vi "L0_Sum.vi"() -> ()   [LabVIEW 2012]
uses:
  <vilib>/Utility/file.llb/Write To Spreadsheet File (string).vi
panel:
  in  "Atenuation":i32[](array[numeric])=[0, 4, 8, 12]
  out "Clip Index":i32=3
  out "Attenuation":i32=12
  out "Ib Clipping\nLevel":i32=63
  in  "Ib Clipping":i32[](array[numeric])=[1, 16, 32, 64, 32, 40, 48, 56, 63]
  out "Delay Line\n(Asic Chan.)":i32=5
  out "VISA resource name out":refnum<visa-resource-name>
  out "error 2 out":errorcluster={"status"=TRUE, "code"=-1073807202, "source"="VISA Open in Agilent 81150.lvlib:Initialize.vi->Set_Gen_Conf.vi->L0_ClippingNDiscrim.vi"}
  in  "error in 1":errorcluster
  in  "Osc":refnum<visa-resource-name>="Oscilloscope"
  in  "Generator":refnum<visa-resource-name>="generadorpulsos"
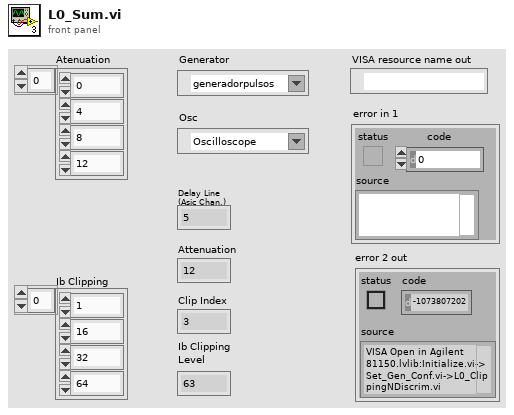
[diagram p1: front panel]
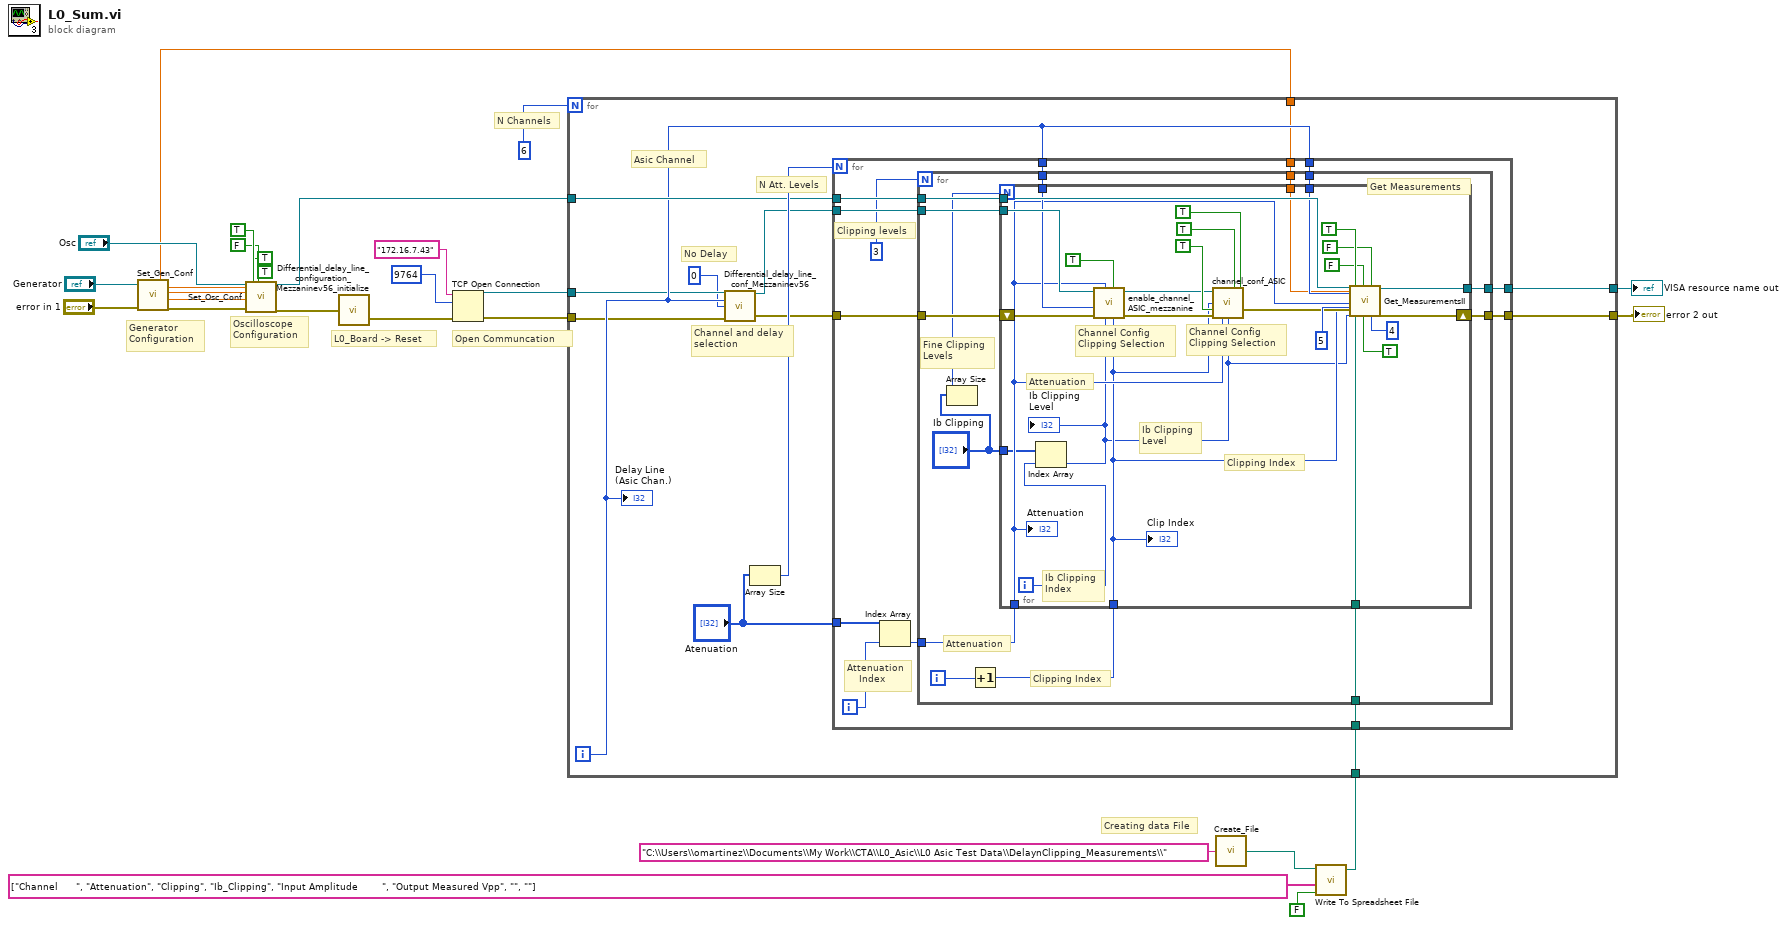
[diagram p0: block diagram]
diagram:
  # "Creating data File"
  # "Open Communcation"
  # "Oscilloscope\nConfiguration"
  # "Generator \nConfiguration"
  # "N Channels"
  # "L0_Board -> Reset"
  n1 = call "Set_Gen_Conf.vi"("AWG VISA"="Generator", "error in (no error)"="error in 1") -> ("Amplitude 1 OUT"=w1:dbl, "Pulse Width in seconds 1 OUT"=w10:dbl, "Trigger Level 1"=w11:dbl, "error out"=w18:errorcluster)  [unwired: 10 in, 4 out]
  n2 = call "Set_Osc_Conf.vi"("VISA resource name"="Osc", "Amplitude IN"=w1, "Trigger Level IN"=w11, "Pulse Width in seconds IN"=w10, "error in (no error)"=w18, "Channel 1"=TRUE, "Channel 3"=TRUE, "Channel 2"=FALSE, "Channel 4"=TRUE) -> ("VISA resource name out"=w6:refnum<visa-resource-name>, "error out"=w17:errorcluster)  [unwired: 9 in]
  n3 = call "Differential_delay_line_configuration_Mezzaninev56_initialize.vi"("error in (no error)"=w17) -> ("error out 2"=w14:errorcluster)  [unwired: 1 in]
  n4 = TCP Open Connection(address="172.16.7.43", remote port or service name=u16 9764, error in (no error)=w14) -> (connection ID=w5:refnum<k5>, error out=w4:errorcluster)  [unwired: 2 in]
  n5 = call "Create_File.vi"("String"="C:\\Users\\omartinez\\Documents\\My Work\\CTA\\L0_Asic\\L0 Asic Test Data\\DelaynClipping_Measurements\\") -> ("path"=w12:path)
  n6 = call-poly <vilib>:"Write To Spreadsheet File.vi"("append to file? (new file:F)"=FALSE, "1D data"=string[] ["Channel      ", "Attenuation", "Clipping", "Ib_Clipping", "Input Amplitude        ", "Output Measured Vpp", "", ""], "file path (dialog if empty)"=w12) -> ("new file path (Not A Path if cancelled)"=w2:path)  [unwired: 5 in]
  n7 = for {
    N: 6 -> [_]
    tunnel: w5 -> [w32]
    tunnel: w4 -> [w33]
    tunnel: w6 -> [w35]
    tunnel: [w29] -> w9
    tunnel: [w30] -> w8
    tunnel: w2 -> [w31]
    tunnel: w1 -> [w27]
    i -> [w34]
    # "No Delay"
    # "Asic Channel"
    # "N Att. Levels"
    # "Channel and delay\nselection"
    n8 = call "Differential_delay_line_conf_Mezzaninev56.vi"("connection ID"=w32, "channel"=w34, "Delay value"=0, "error in (no error)"=w33) -> ("connection ID out"=w36:refnum<k5>, "error out 2"=w37:errorcluster)  [unwired: 4 in, 6 out]
    n9 = Array Size(array="Atenuation") -> (size(s)=w38:i32)
    n10 = for {
      N: w38 -> [_]
      tunnel: w36 -> [w52]
      tunnel: w35 -> [w51]
      tunnel: w37 -> [w50]
      tunnel: "Atenuation" -> [w48]
      tunnel: w34 -> [w45]
      tunnel: w31 -> [w44]
      tunnel: w34 -> [w43]
      tunnel: [w42] -> w29
      tunnel: [w41] -> w30
      tunnel: w27 -> [w40]
      i -> [w47]
      # "Clipping levels"
      # "Attenuation\n    Index"
      n11 = Index Array(array=w48, index=w47) -> (element=w46:i32)
      n12 = for {
        N: 3 -> [_]
        tunnel: w52 -> [w66]
        tunnel: w51 -> [w65]
        tunnel: w50 -> [w64]
        tunnel: w46 -> [w61]
        tunnel: w45 -> [w62]
        tunnel: w44 -> [w59]
        tunnel: w43 -> [w58]
        tunnel: [w57] -> w42
        tunnel: [w56] -> w41
        tunnel: w40 -> [w53]
        i -> [w63]
        # "Get Measurements"
        # "Fine Clipping\nLevels"
        # "Attenuation"
        # "Clipping Index"
        n13 = Array Size(array="Ib Clipping") -> (size(s)=w55:i32)
        n14 = Increment(x=w63) -> (x+1=w60:i32)
        n15 = for {
          N: w55 -> [_]
          tunnel: w66 -> [w90]
          tunnel: w65 -> [w86]
          tunnel: w61 -> [w74]
          tunnel: w62 -> [w84]
          tunnel: w60 -> [w73]
          tunnel: w59 -> [w82]
          tunnel: w58 -> [w80]
          tunnel: [w77] -> w56
          shift-right: [w78] -> w57
          shift-left: w64 -> [w85]
          tunnel: "Ib Clipping" -> [w72]
          tunnel: w53 -> [w69]
          i -> [w70]
          # "Channel Config\nClipping Selection"
          # "Clipping Index"
          # "Ib Clipping\nLevel"
          # "Attenuation"
          # "Ib Clipping\nIndex"
          # "Channel Config\nClipping Selection"
          n16 = Index Array(array=w72, index=w70) -> (element=w71:i32)
          "Ib Clipping\nLevel" <- w71
          n17 = call "enable_channel_ASIC_mezzanine.vi"("Clip_sel_b"=w73, "maj/sum"=TRUE, "Ib_clipVb"=w71, "Att gain"=w74, "error in"=w85, "Channel"=w84, "connection ID"=w90) -> ("error out"=w91:errorcluster, "connection ID out"=w89:refnum<k5>)  [unwired: 2 in, 1 out]
          n18 = call "channel_conf_ASIC.vi"("connection ID"=w89, "Clip_sel_b"=w73, "CompBuf_en_b"=TRUE, "error out"=w91, "Att gain"=w74, "Ib_ClipVb"=w71, "Clip_en_b"=TRUE, "Att_en_b"=TRUE) -> ("error out 2"=w75:errorcluster)  [unwired: 3 in, 4 out]
          n19 = call "Get_MeasurementsII.vi"("VISA resource name"=w86, "Amplitude IN"=w69, "Attenuation"=w74, "Measurements per channel"=5, "Clipping"=w73, "Fine Clipping"=w71, "Amplitude"=TRUE, "file path (dialog if empty)"=w82, "Width"=FALSE, "Write to a file?"=TRUE, "ASIC Channel"=w80, "error in"=w75, "Delay"=FALSE, "Oscilloscope Channel"=4) -> ("VISA resource name out"=w77:refnum<visa-resource-name>, "error out"=w78:errorcluster)  [unwired: 9 in, 3 out]
          "Clip Index" <- w73
          "Attenuation" <- w74
        }
      }
    }
    "Delay Line\n(Asic Chan.)" <- w34
  }
  "error 2 out" <- w9
  "VISA resource name out" <- w8
